vi "Peregrine_I2C_read.vi"(0 "Handle in":refnum<visa-resource-name>, 2 "Address":u8, 5 "i2c address":u32, 11 "error":errorcluster) -> (4 "Handle out":refnum<visa-resource-name>, 6 "Key response":u32, 8 "Value response":i32, 15 "error out":errorcluster)   [LabVIEW 2019]
panel:
  out "Command":i32
  out "Address response":u8
  # "Inputs"
  # "Response message"
  # "Output"
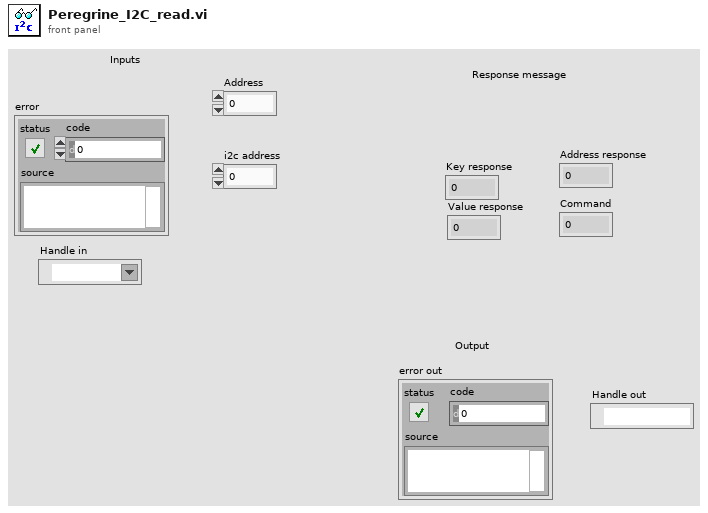
[diagram p1: front panel]
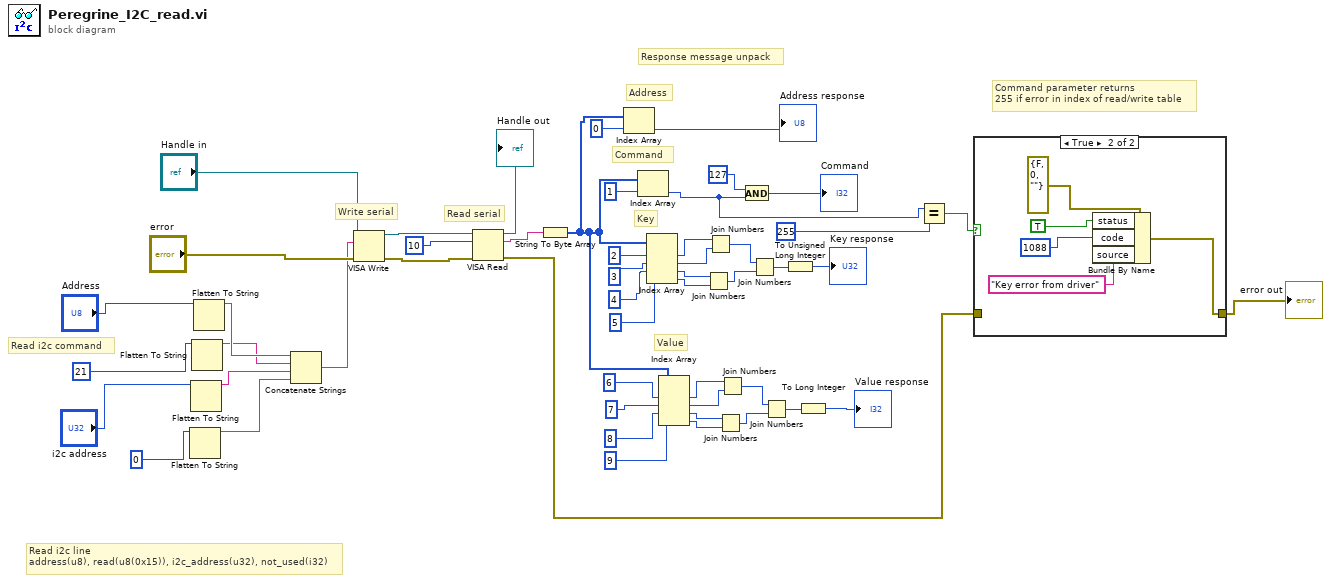
[diagram p0: block diagram]
diagram:
  # "Command parameter returns\n255 if error in index of read/write table"
  # "Value"
  # "Response message unpack"
  # "Read i2c command"
  # "Command"
  # "Address"
  # "Key"
  # "Read serial"
  # "Write serial"
  # "Read i2c line\naddress(u8), read(u8(0x15)), i2c_address(u32), not_used(i32)"
  n1 = Flatten To String(anything=0) -> (data string=w25:string)  [unwired: 3 in, 2 out]
  n2 = Flatten To String(anything="i2c address") -> (data string=w26:string)  [unwired: 3 in, 2 out]
  n3 = Flatten To String(anything=u8 21) -> (data string=w2:string)  [unwired: 3 in, 2 out]
  n4 = Flatten To String(anything="Address") -> (data string=w28:string)  [unwired: 3 in, 2 out]
  n5 = Concatenate Strings(w28, w2, w26, w25) -> (w1:string)
  n6 = VISA Write(VISA resource name="Handle in", write buffer=w1, error in (no error)="error") -> (VISA resource name out=w51:refnum<visa-resource-name>, error out=w30:errorcluster)  [unwired: 1 out]
  n7 = VISA Read(VISA resource name=w51, byte count=10, error in (no error)=w30) -> (VISA resource name out=→"Handle out":refnum<visa-resource-name>, read buffer=w49:string, error out=w6:errorcluster)  [unwired: 1 out]
  n8 = String To Byte Array(string=w49) -> (unsigned byte array=w16:u8[])
  n9 = Index Array(array=w16, index=0) -> (element=→"Address response":u8)
  n10 = Index Array(array=w16, index=1) -> (element=w9:u8)
  n11 = Index Array(array=w16, index #1=2, index #2=3, index #3=4, index #4=5) -> (element #1=w42:u8, element #2=w41:u8, element #3=w40:u8, element #4=w39:u8)
  n12 = Index Array(array=w16, index #1=6, index #2=7, index #3=8, index #4=9) -> (element #1=w23:u8, element #2=w22:u8, element #3=w21:u8, element #4=w20:u8)
  n13 = Join Numbers(hi=w40, lo=w39) -> ((hi.lo)=w38:u16)
  n14 = Join Numbers(hi=w42, lo=w41) -> ((hi.lo)=w37:u16)
  n15 = Join Numbers(hi=w21, lo=w20) -> ((hi.lo)=w19:u16)
  n16 = Join Numbers(hi=w23, lo=w22) -> ((hi.lo)=w18:u16)
  n17 = And(x=127, y=w9) -> (x .and. y?=→"Command":i32)
  n18 = Join Numbers(hi=w37, lo=w38) -> ((hi.lo)=w11:u32)
  n19 = Join Numbers(hi=w18, lo=w19) -> ((hi.lo)=w12:u32)
  n20 = To Unsigned Long Integer(number=w11) -> (unsigned 32bit integer=→"Key response":u32)
  n21 = To Long Integer(number=w12) -> (32bit integer=→"Value response":i32)
  n22 = Equal?(x=w9, y=255) -> (x = y?=w7:bool)
  n23 = case shown="True" w7 {
    tunnel: w6 -> [w52 _]
    tunnel: [w52 w54] -> w5
    frame False {
    }
    frame True {
      n24 = Bundle By Name(cluster=errorcluster {"status"=FALSE, "code"=0, "source"=""} ("error constant"), "status"=TRUE, "code"=1088, "source"="Key error from driver") -> (w54:errorcluster)
    }
  }
  "error out" <- w5
